vi "DefineScan.vi"() -> ()   [LabVIEW 2011]
doc: "Element for defineing the region to scan"
uses:
  <vilib>/vision/NI_Vision_Development_Module.lvlib
panel:
  out "Galvo pos i.image [m]":cluster{dbl, dbl}={0.005744, 0.00027999999999999987} {"?" format="%#_3p"; "?" format="%#_3p"}
  in  "Registerkarte":enum32{"scan", "view", "option"}(tab)
  in  "experiment":string="mysample_01"
  in  "pixels":cluster{"x-Pixel":i32, "y-Pixel":u16}={"x-Pixel"=400, "y-Pixel"=400} {"y-Pixel" min=2 max=4000 step=2; "x-Pixel" min=10 max=4000 step=1}
  in  "keep const.":u16(ring) items=["pix. size", "pixels"]
  in  "pixel size":cluster{dbl, dbl}={3e-07, 3e-07} {"?" min=0.0 max=0.01 step=5e-08 format="%#_4p"; "?" min=0.0 max=0.01 step=5e-08 format="%#_4p"}
  out "Turn loss %":dbl=0.5000000000000115 format="%#_4f"
  out "total time [s]":dbl=1.6 min=0.0005 step=0.001 format="%#_3f"
  in  "image size [m]":cluster{"x":dbl, "y":dbl}={"x"=0.00012, "y"=0.00012} {"y" min=0.0 max=0.01 step=1e-06 format="%#_4p"; "x" min=0.0 max=0.01 step=1e-06 format="%#_4p"}
  in  "Bidirektional":bool=TRUE
  in  "time [s]/point":dbl=1e-05 min=2.5e-07 step=1e-06 format="%#_3p"
  in  "ChangeScan":bool
  in  "Maximum":i32=97
  in  "Minimum":i32=3
  in  "Image loading method":bool=TRUE caption="Scan          calibration(new)"
  in  "Image to load":enum16{"marked", "last", "penultimate", "clear"}(ring)
  in  "scan to load":enum16{"marked", "last", "active"}(ring)=enum."last"
  in  "Galvo center [m] ii":cluster{dbl, dbl}={0.0002, -0.0008} {"?" min=-0.1 max=0.1 step=0.0001; "?" min=-0.1 max=0.1 step=0.0001}
  in  "LoadNewScan":bool
  in  "radius of view-x (6m)":dbl=0.006 min=0.0005 max=0.1 step=0.001
  in  "LoadNewImage":bool
  in  "Display Mapping Method":u32(ring)=16 items=["Default"=10, "Most Significant Bits"=11, "Full Dynamic"=12, "Downshift"=13, "Given Range"=14, "90% Dynamic"=15, "Given Percent Range"=16]
  in  "Image Oversampling":sgl=1.0 min=0.5 max=10 step=1
  in  "parabolic turn":bool=TRUE
  in  "times higher accelaration":dbl=1.0 min=1e-06 max=1000000.0 step=0.05
  in  "Transform":T1={"00 Pixel [m]"={-0.0058000000000000005, 0.0052}, "Rotate (rad)"=-0.0, "MirrorY"=TRUE, "pix/m"=41666.666666666664} caption="Pixel>Scan-i.image[m]" {"00 Pixel [m]"."?" format="%#_3p"; "00 Pixel [m]"."?" format="%#_3p"}
  in  "galvorotation (grad)":dbl=-0.0
  out "galvocycle":dbl=1e-05
  out "adclock":dbl=4000000.0
  in  "Objektive":dbl=60.0 format="%.1f"
  in  "SMdelay [Cycles]":i16=119
  in  "do not close at end":bool
  out "Image":T2(plugin-control)
  in  "Exit":bool
  # "m for 1E-3\nu for 1E-6\nn for 1E-9"
  # "all referenced to\nintermediate image\n!! so far no update: load new!"
  # "real position is \ni.image*Maginfication"
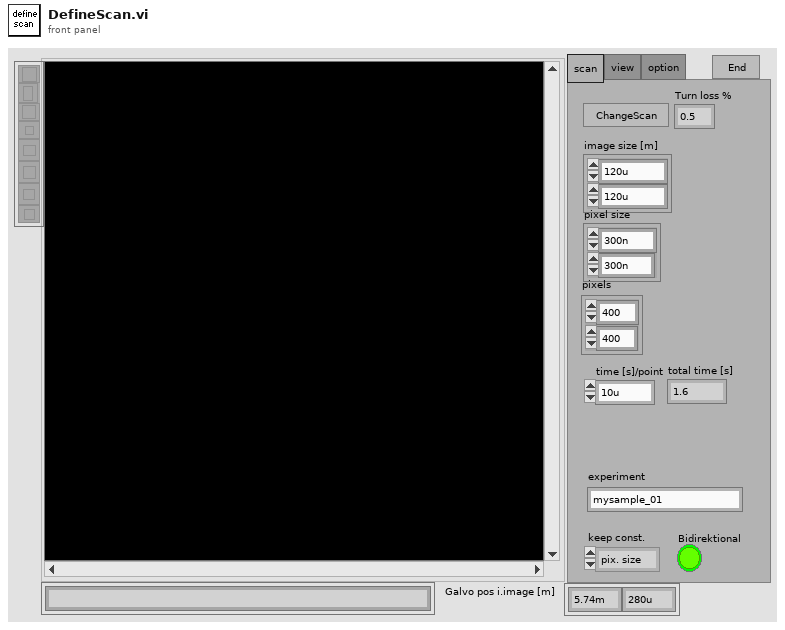
[diagram p1: front panel]
types:
  T1 = cluster{"00 Pixel [m]":cluster{dbl, dbl}, "Rotate (rad)":dbl, "MirrorY":bool, "pix/m":dbl}
  T2 = typedef "IMAQ Image.ctl" = refnum<image>
  T3 = cluster{"Pixel":i32, "Smartmovedelay [s]":dbl, "Loops":i32, "Bidirektional":bool, "SMCycle [s]":dbl, "AD-Frequency [Hz]":dbl, "Grad/m":dbl}
  T4 = typedef "Image Type" = u32
  T5 = enum16{"None/#Datasets", "Clear", "TagValueOf#", "AddValues", "ReadValue", "ChangeValue", "Get all"}
  T6 = cluster{"x Pixel":i32, "Lines":i32, "Bidirektional":bool, "AD-Frequency [Hz]":dbl, "Galvo Cycle [s]":dbl, "Galvodelay [s]":dbl, "max.accel. [m/s^2]":dbl}
  T7 = cluster{"Pixel":i32, "Smartmovedelay [s]":dbl, "lines":i32, "Bidirektional":bool, "SMCycle [s]":dbl, "AD-Frequency [Hz]":dbl, "Grad/m":dbl}
  T8 = cluster{"Zeit/Spirale (sync Pixel)":dbl, "Center":cluster{"x":dbl, "y":dbl}, "Radius":dbl}
  T9 = cluster{"Pixel on spiral":i32, "Smartmovedelay [s]":dbl, "lines":i32, "Bidirektional":bool, "SMCycle [s]":dbl, "AD-Frequency [Hz]":dbl, "Grad/m":dbl}
  T10 = typedef "Image Unit" = enum32{"Undefined", "Angström", "Micrometer", "Millimeter", "Centimeter", "Meter", "Kilometer", "Microinch", "Inch", "Feet", "Nautical miles", "Standard miles", "Steps"}
  T11 = enum16{"status", "createIMAQ", "getIMAQ", "getNumber", "deleteIMAQ", "deleteAll", "MemoryUsage", "GetAccess", "DecreaseAccess", "ActualIndex", "ElementToNumber"}
  T12 = enum16{"status", "saveMeta", "getMeta", "deleteMeta", "deleteAll", "MemoryUsage"}
  T13 = cluster{"Global Rectangle":i32[], "Contours":cluster{"Contour Type":u32, "ROI Type":u32, "Points":i32[]}[]}
  T14 = cluster{"Contour Type":u32, "ROI Type":u32, "Points":i32[]}[]
  T15 = cluster{"Contour Type":u32, "ROI Type":u32, "Points":i32[]}
  T16 = typedef "ScanControl.ctl" = cluster{"Time [s]":dbl, "action":T17, "channel":T18, "value (/s)":dbl}[]
  T17 = typedef "ScanControl_Action.ctl" = enum16{"Abs", "Rel", "Inc", "IncInc", "LoopStart", "LoopEnd", "WaitTriggerRising"}
  T18 = typedef "ScanControl_Channel.ctl" = enum16{"Com", "AnalogConfig", "AnalogValue", "GalvoX", "GalvoY", "Galvo3", "Galvo4", "Digital", "Free", "Loop", "SMoveTime", "Image1X", "Image1Y", "Image2X", "Image2Y"}
  T19 = cluster{"Global Rectangle[0]":i32, "Global Rectangle[1]":i32}
  T20 = cluster{"Point Out":cluster{dbl, dbl}, cluster{dbl, dbl}, cluster{dbl, dbl}, dbl}
  T21 = cluster{"Zeitpunkt [s]":dbl, "Wirkung":enum16{"Abs", "Rel", "Inc", "IncInc", "LoopStart", "LoopEnd"}, "Kanal":enum16{"Com", "AnalogConfig", "AnalogValue", "GalvoX", "GalvoY", "Galvo3", "Galvo4", "Digital", "Free", "Loop", "SMoveTime", "Image1X", "Image1Y", "Image2X", "Image2Y"}, "Wert (/s)":dbl}[]
  T22 = cluster{"fast/slow [m(ii)][0]":cluster{"x":dbl, "y":dbl}, "fast/slow [m(ii)][1]":cluster{"x":dbl, "y":dbl}}
  T23 = cluster{"number: 0 to 1":dbl, "number: 0 to 1":dbl}[]
  T24 = cluster{i32[], cluster{"Contour Type":u32, "ROI Type":u32, i32[]}[]}
  T25 = cluster{"Contour Type":u32, "ROI Type":u32, i32[]}[]
  T26 = cluster{"Contour Type":u32, "ROI Type":u32, i32[]}
  T27 = cluster{"Global Rectangle[0]":i32, "Global Rectangle[1]":i32, "Global Rectangle[2]":i32, "Global Rectangle[3]":i32}
  T28 = cluster{"Global Rectangle[2]":i32, "Global Rectangle[3]":i32}
  T29 = cluster{"Points[0]":i32, "Points[1]":i32, "Points[2]":i32, "Points[3]":i32, "Points[4]":i32}
  T30 = cluster{"Points[0]":i32, "Points[1]":i32, "Points[2]":i32, "Points[3]":i32}
  T31 = cluster{i32[], cluster{"Contour Type":u32, "ROI Type":u32, "Points":i32[]}[]}
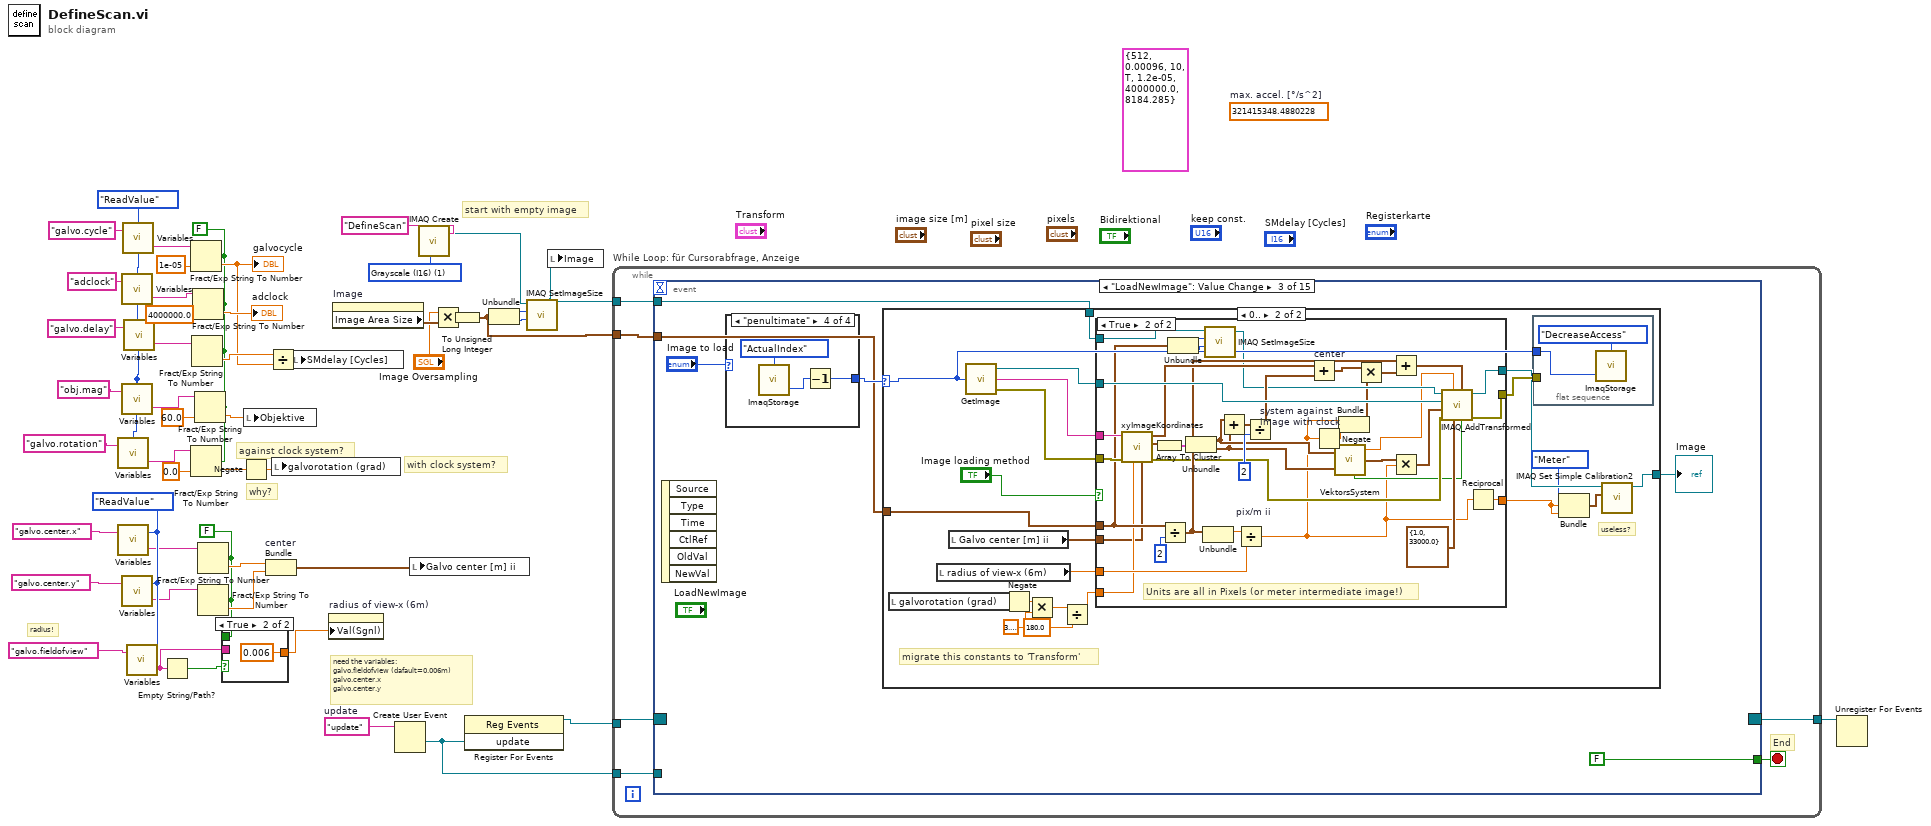
[diagram p0: block diagram]
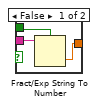
[diagram p2: hidden frame]
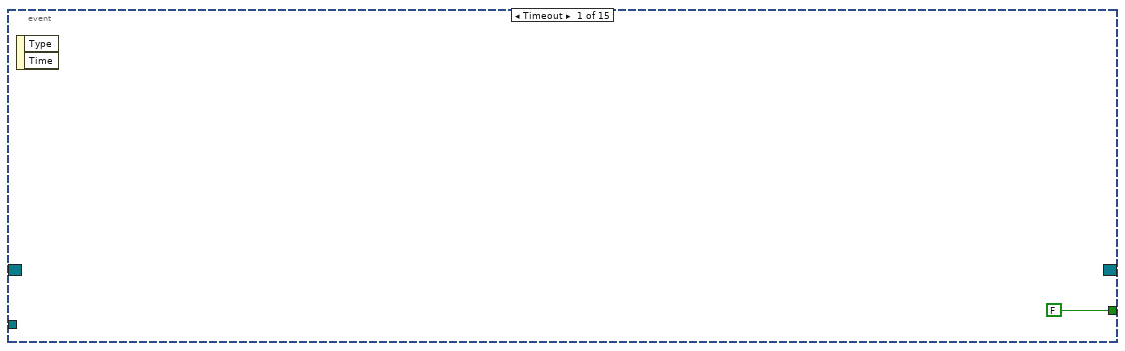
[diagram p3: hidden frame]
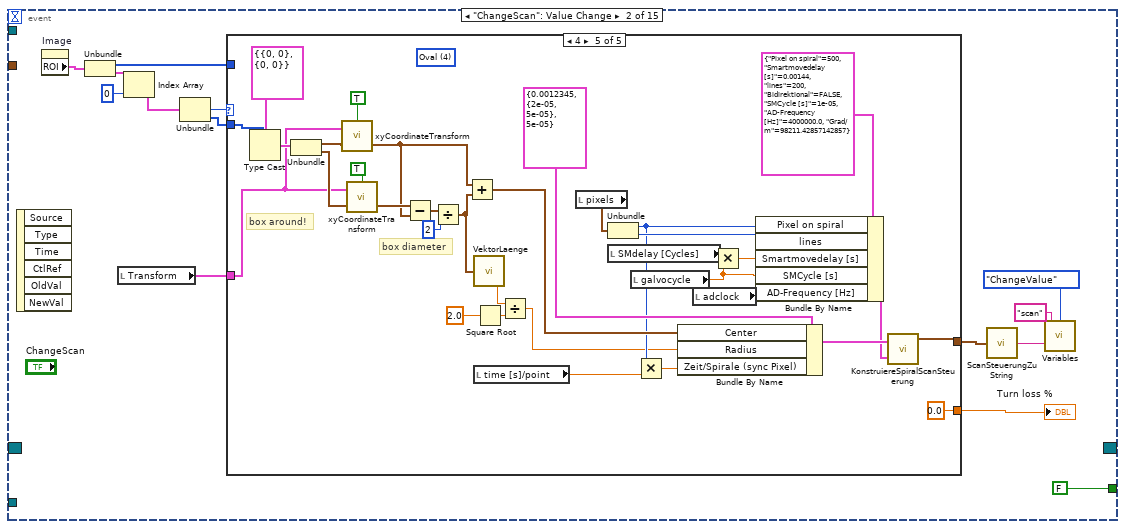
[diagram p4: hidden frame]
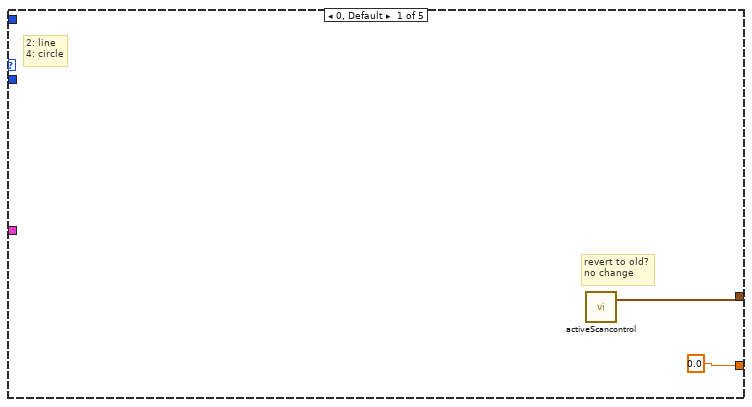
[diagram p5: hidden frame]
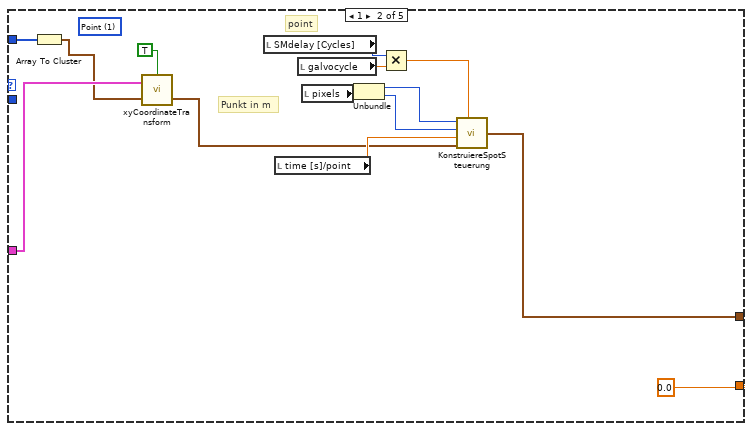
[diagram p6: hidden frame]
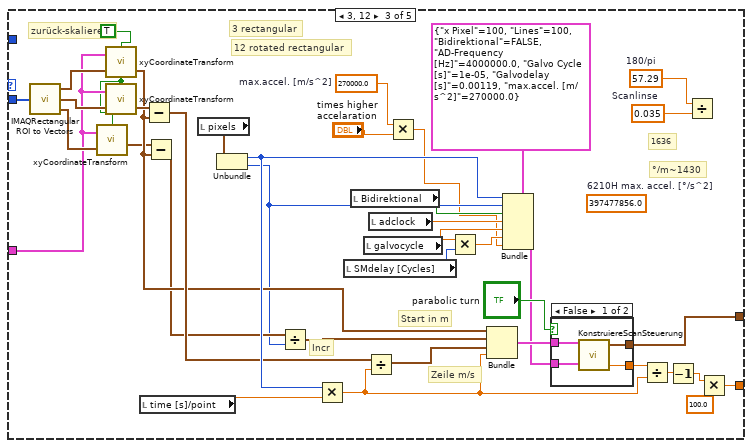
[diagram p7: hidden frame]
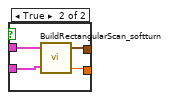
[diagram p8: hidden frame]
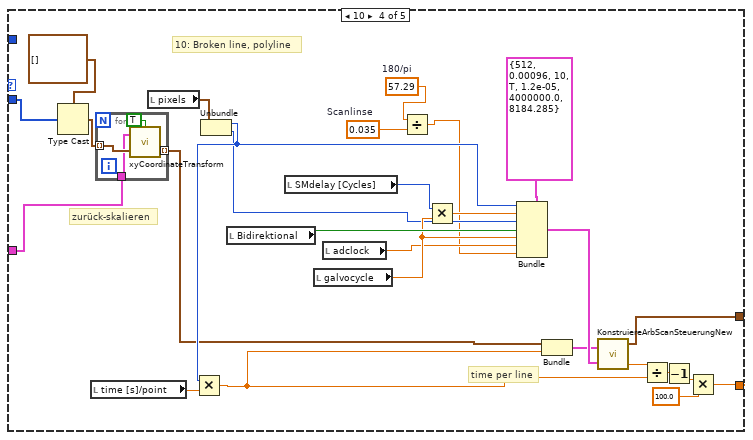
[diagram p9: hidden frame]
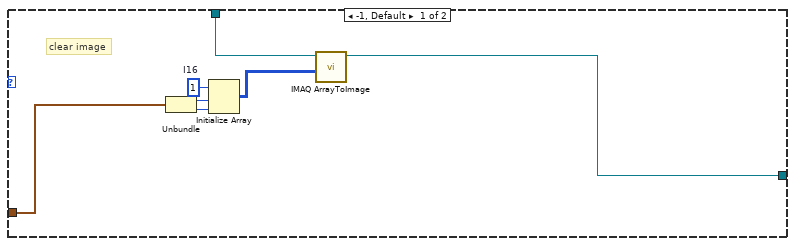
[diagram p10: hidden frame]
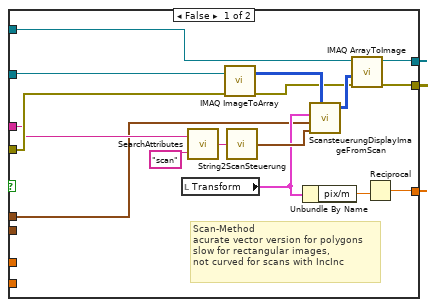
[diagram p11: hidden frame]
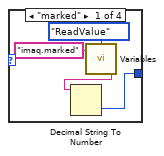
[diagram p12: hidden frame]
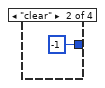
[diagram p13: hidden frame]
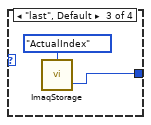
[diagram p14: hidden frame]
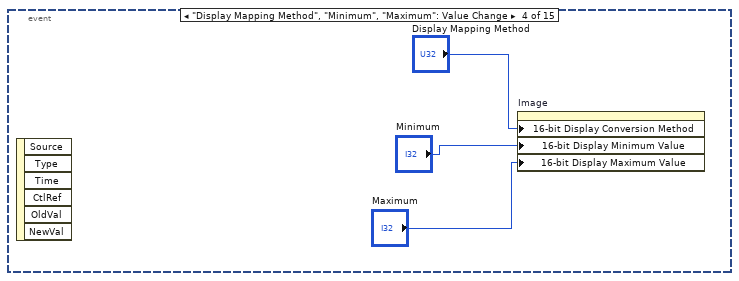
[diagram p15: hidden frame]
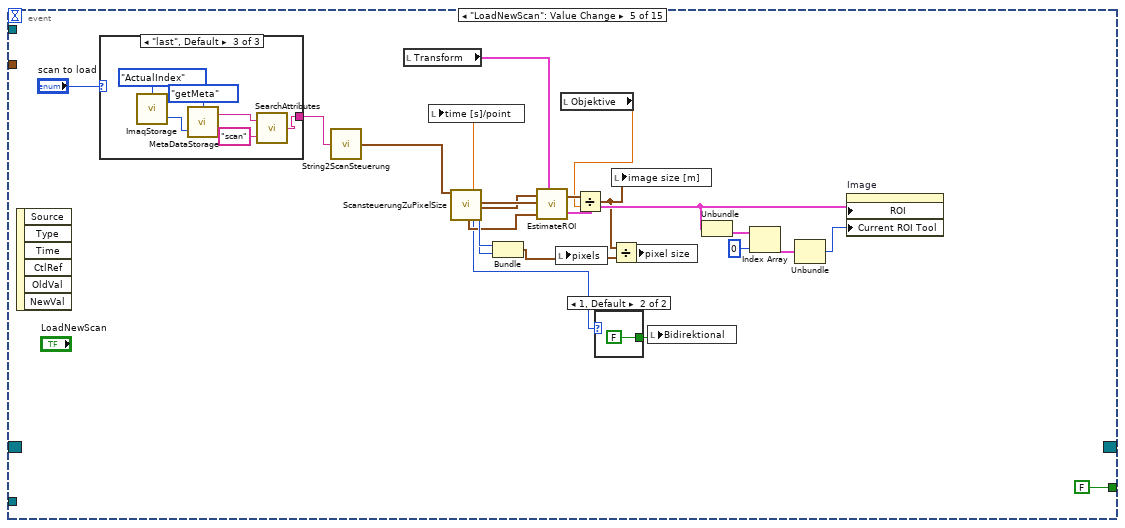
[diagram p16: hidden frame]
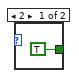
[diagram p17: hidden frame]
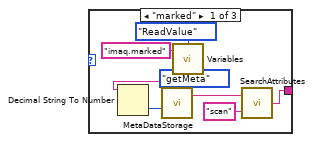
[diagram p18: hidden frame]
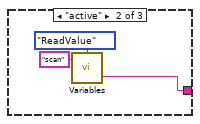
[diagram p19: hidden frame]
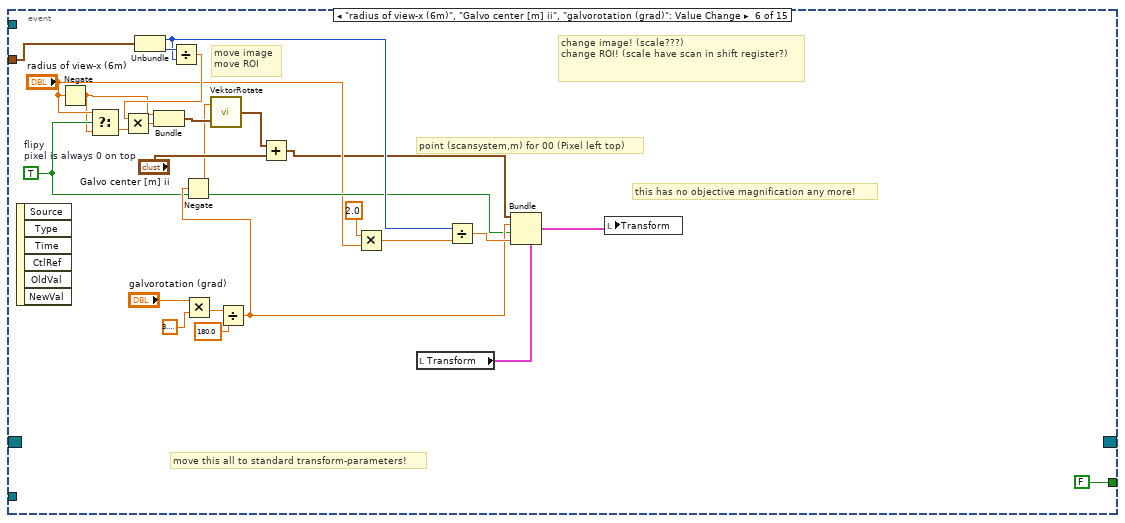
[diagram p20: hidden frame]
diagram:
  (unwired) 321415348.4880228  # max. accel. [°/s^2]
  (unwired) T3 {"Pixel"=512, "Smartmovedelay [s]"=0.00096, "Loops"=10, "Bidirektional"=TRUE, "SMCycle [s]"=1.2e-05, "AD-Frequency [Hz]"=4000000.0, "Grad/m"=8184.285} ("ParameterCluster")
  w10 = T4 1 items=["Grayscale (U8)", "Grayscale (I16)", "Grayscale (SGL)", "Complex (CSG)", "RGB (U32)", "HSL (U32)", "RGB (U64)", "Grayscale (U16)"] ("Image Type")
  w27 = FALSE ("use system decimal point (T)")
  w26 = T5."ReadValue" ("Command")
  w39 = "update"  # update
  w15 = FALSE ("use system decimal point (T)")
  w14 = T5."ReadValue" ("Command")
  # "against clock system?"
  # "with clock system?"
  # "why?"
  # "start with empty image"
  # "radius!"
  # "need the variables:\ngalvo.fieldofview (dafault=0.006m)\ngalvo.center.x\ngalvo.center.y"
  n1 = call "Variables.vi"("Tag in"="galvo.rotation", "Command"=w14) -> ("value out"=w17:string)  [unwired: 1 in, 2 out]
  n2 = call "Variables.vi"("Tag in"="galvo.center.x", "Command"=w26) -> ("value out"=w24:string)  [unwired: 1 in, 2 out]
  n3 = call "Variables.vi"("Tag in"="adclock", "Command"=w14) -> ("value out"=w47:string)  [unwired: 1 in, 2 out]
  n4 = call "Variables.vi"("Tag in"="obj.mag", "Command"=w14) -> ("value out"=w43:string)  [unwired: 1 in, 2 out]
  n5 = call "Variables.vi"("Tag in"="galvo.center.y", "Command"=w26) -> ("value out"=w23:string)  [unwired: 1 in, 2 out]
  n6 = call "Variables.vi"("Tag in"="galvo.cycle", "Command"=w14) -> ("value out"=w46:string)  [unwired: 1 in, 2 out]
  n7 = call "Variables.vi"("Tag in"="galvo.delay", "Command"=w14) -> ("value out"=w35:string)  [unwired: 1 in, 2 out]
  n8 = call "Variables.vi"("Tag in"="galvo.fieldofview", "Command"=w26) -> ("value out"=w30:string)  [unwired: 1 in, 2 out]
  n9 = Empty String/Path?(string/path=w30) -> (empty?=w31:bool)
  n10 = Fract/Exp String To Number(use system decimal point (T)=w15, string=w46, default (0 dbl)=1e-05 ("default (0 DBL)")) -> (number=w33:dbl)  [unwired: 2 out]
  "galvocycle" <- w33
  n11 = Fract/Exp String To Number(use system decimal point (T)=w15, string=w17, default (0 dbl)=0.0 ("default (0 DBL)")) -> (number=w13:dbl)  [unwired: 2 out]
  n12 = Fract/Exp String To Number(use system decimal point (T)=w15, string=w35) -> (number=w34:dbl)  [unwired: 3 out]
  n13 = Fract/Exp String To Number(use system decimal point (T)=w15, string=w47, default (0 dbl)=4000000.0 ("default (0 DBL)")) -> (number=→"adclock":dbl)  [unwired: 2 out]
  n14 = Fract/Exp String To Number(use system decimal point (T)=w15, string=w43, default (0 dbl)=60.0 ("default (0 DBL)")) -> (number=w20:dbl)  [unwired: 2 out]
  n15 = Fract/Exp String To Number(use system decimal point (T)=w27, string=w24) -> (number=w28:dbl)  [unwired: 3 out]
  n16 = Fract/Exp String To Number(use system decimal point (T)=w27, string=w23) -> (number=w29:dbl)  [unwired: 3 out]
  n17 = case shown="True" w31 {
    tunnel: w30 -> [w53 _]
    tunnel: w27 -> [w52 _]
    tunnel: [w51 0.006] -> w11
    frame False {
      n18 = Fract/Exp String To Number(use system decimal point (T)=w52, string=w53) -> (number=w51:dbl)  [unwired: 3 out]
    }
    frame True {
    }
  }
  n19 = Negate(x=w13) -> (-x=w12:dbl)
  n20 = local write "Objektive"(w20) -> ()
  n21 = Bundle "center"(w28, w29) -> (w19:cluster{dbl, dbl})  [unwired: 1 out]
  n22 = Divide(x=w34, y=w33) -> (x/y=w32:dbl)
  n23 = local write "galvorotation (grad)"(w12) -> ()
  n24 = local write "SMdelay [Cycles]"(w32) -> ()
  n25 = property on="radius of view-x (6m)" class="DigNum (strict)"("Val(Sgnl)"=w11) -> ()  [unwired: 2 in, 2 out]
  n26 = property on="Image" class="ImageControl"() -> ("Image Area Size"=w6:cluster{"Width":u32, "Height":u32})  [unwired: 2 in, 2 out]
  n27 = Create User Event(user event datatype=w39) -> (user event=w36:refnum<user-event>)  [unwired: 1 in, 1 out]
  n28 = local write "Galvo center [m] ii"(w19) -> ()
  n29 = call "IMAQ Create"("Image Name"="DefineScan", "Image Type"=w10) -> ("New Image"=w5:T2)  [unwired: 2 in, 2 out]
  n30 = Multiply(x="Image Oversampling", y=w6) -> (x*y=w3:cluster{"Width":sgl, "Height":sgl})
  n31 = To Unsigned Long Integer(number=w3) -> (unsigned 32bit integer=w1:cluster{"Width":u32, "Height":u32})
  n32 = register-events(w36) -> (reference out=w38:refnum<event-registration>)  [unwired: 2 in, 1 out]
  n33 = Unbundle(w1) -> ("Width"=w8:u32, "Height"=w7:u32)
  n34 = call "IMAQ SetImageSize"("Y Resolution"=w7, "X Resolution"=w8, "Image"=w5) -> ("Image Out"=w4:T2)  [unwired: 1 in, 2 out]
  n35 = local write "Image"(w4) -> ()
  n36 = while "While Loop: für Cursorabfrage, Anzeige" {
    tunnel: w38 -> [w59]
    tunnel: [w58] -> w37
    tunnel: w36 -> [w57]
    tunnel: w4 -> [w56]
    tunnel: w1 -> [w55]
    stop <- w60 stop-if-true
    # "End"
    n37 = event shown="[2] \"LoadNewImage\": Value Change" {
      selector: w59 -> [_ _ _ _ _ _ _ _ _ _ _ _ _ _ _]
      dyn-events: [_ _ _ _ _ _ _ _ _ _ _ _ _ _ _] -> w58
      timeout: _ -> [_ _ _ _ _ _ _ _ _ _ _ _ _ _ _]
      tunnel: [FALSE FALSE FALSE _ FALSE ("Exit") FALSE ("Exit") FALSE ("Exit") FALSE ("Exit") _ FALSE ("Exit") FALSE ("Exit") FALSE ("Exit") _ "Exit" FALSE] -> w60
      tunnel: w57 -> [_ _ _ _ _ _ _ w385 _ w403 w501 w521 _ _ _]
      tunnel: w56 -> [_ _ w205 _ _ _ _ _ _ _ _ _ _ _ _]
      tunnel: w55 -> [_ _ w202 _ _ w346 _ _ _ _ _ _ _ _ _]
      event Timeout {
        n38 = event-data() -> ()  [unwired: 3 out]
      }
      event "ChangeScan": Value Change {
        n39 = event-data() -> ()  [unwired: 7 out]
        n40 = property on="Image" class="ImageControl"() -> ("ROI"=w74:T13)  [unwired: 2 in, 2 out]
        n41 = Unbundle(w74) -> ("Global Rectangle"=w73:i32[], "Contours"=w72:T14)
        n42 = local read "Transform"() -> (w62:T1)
        n43 = Index Array(array=w72, index=0) -> (element=w70:T15)
        n44 = Unbundle(w70) -> ("ROI Type"=w69:u32, "Points"=w68:i32[])  [unwired: 1 out]
        n45 = case shown="4" w69 {
          tunnel: w73 -> [_ w90 _ _ _]
          tunnel: w68 -> [_ _ w126 w147 w197]
          tunnel: [w77 w87 w118 w151 w201] -> w67
          tunnel: [0.0 0.0 w117 w146 0.0] -> w63
          tunnel: w62 -> [_ w80 w106 w141 w179]
          frame 0, Default {
            # "2: line\n4: circle"
            # "revert to old?\nno change"
            n46 = call "activeScancontrol.vi"() -> ("ScanSteuerung"=w77:T16)  [unwired: 2 in, 1 out]
          }
          frame 1 {
            (unwired) u32 1 items=["No Selection", "Point", "Line", "Rectangle", "Oval", "Polygon", "Free", "Annulus", "Unused2", "Unused3", "Broken Line", "Free Hand Line", "Rotated Rectangle"] ("Type")
            # "Punkt in m"
            # "point"
            n47 = Array To Cluster(array=w90) -> (cluster=w79:T19)
            n48 = call "xyCoordinateTransform.vi"("Point in"=w79, "Transform (Center first)"=w80, "Back"=TRUE) -> ("Point Out"=w78:cluster{dbl, dbl})  [unwired: 2 out]
            n49 = local read "SMdelay [Cycles]"() -> (w91:i16)
            n50 = local read "time [s]/point"() -> (w88:dbl)
            n51 = local read "galvocycle"() -> (w86:dbl)
            n52 = local read "pixels"() -> (w84:cluster{"x-Pixel":i32, "y-Pixel":u16})
            n53 = Unbundle(w84) -> ("x-Pixel"=w83:i32, "y-Pixel"=w82:u16)
            n54 = Multiply(x=w91, y=w86) -> (x*y=w89:dbl)
            n55 = call "KonstruiereSpotSteuerung.vi"("SMtime"=w89, "Punkt [m]"=w78, "Time [s]/Point"=w88, "y-Pixel"=w82, "x-Pixel"=w83) -> ("ScanSteuerung"=w87:T16)  [unwired: 1 out]
          }
          frame 3, 12 {
            w94 = 270000.0  # max.accel. [m/s^2]
            (unwired) 397477856.0  # 6210H max. accel. [°/s^2]
            w105 = TRUE ("Back")
            w104 = 57.29  # 180/pi
            w129 = 0.035  # Scanlinse
            # "°/m~1430"
            # "1636"
            # "3 rectangular"
            # "12 rotated rectangular"
            # "Start in m"
            # "zurück-skalieren"
            # "Zeile m/s"
            # "Incr"
            n56 = call "IMAQRectangularROI to Vectors.vi"("Array"=w126) -> ("Start"=w114:cluster{"x":dbl, "y":dbl}, "fast end"=w113:cluster{"x":dbl, "y":dbl}, "slow end"=w111:cluster{"x":dbl, "y":dbl})
            n57 = call "xyCoordinateTransform.vi"("Point in"=w111, "Transform (Center first)"=w106, "Back"=w105) -> ("Point Out"=w108:cluster{dbl, dbl})  [unwired: 2 out]
            n58 = call "xyCoordinateTransform.vi"("Point in"=w114, "Transform (Center first)"=w106, "Back"=w105) -> ("Point Out"=w109:cluster{dbl, dbl})  [unwired: 2 out]
            n59 = call "xyCoordinateTransform.vi"("Point in"=w113, "Transform (Center first)"=w106, "Back"=w105) -> ("Point Out"=w110:cluster{dbl, dbl})  [unwired: 2 out]
            n60 = local read "time [s]/point"() -> (w127:dbl)
            n61 = Subtract(x=w110, y=w109) -> (x-y=w112:cluster{dbl, dbl})
            n62 = Subtract(x=w108, y=w109) -> (x-y=w107:cluster{dbl, dbl})
            n63 = local read "pixels"() -> (w116:cluster{"x-Pixel":i32, "y-Pixel":u16})
            n64 = Unbundle(w116) -> ("x-Pixel"=w115:i32, "y-Pixel"=w100:u16)
            n65 = Divide(x=w107, y=w100) -> (x/y=w125:cluster{dbl, dbl})
            n66 = Multiply(x=w115, y=w127) -> (x*y=w122:dbl)
            n67 = local read "SMdelay [Cycles]"() -> (w95:i16)
            n68 = local read "Bidirektional"() -> (w99:bool)
            n69 = local read "galvocycle"() -> (w96:dbl)
            n70 = Divide(x=w112, y=w122) -> (x/y=w124:cluster{dbl, dbl})
            n71 = local read "adclock"() -> (w98:dbl)
            n72 = Multiply(x=w94, y="times higher accelaration") -> (x*y=w92:dbl)
            n73 = Multiply(x=w96, y=w95) -> (x*y=w97:dbl)
            n74 = Bundle("Point Out"=w109, w125, w124, w122) -> (w128:T20)  [unwired: 1 out]
            n75 = Bundle(cluster=T6 {"x Pixel"=100, "Lines"=100, "Bidirektional"=FALSE, "AD-Frequency [Hz]"=4000000.0, "Galvo Cycle [s]"=1e-05, "Galvodelay [s]"=0.00119, "max.accel. [m/s^2]"=270000.0} ("ParameterCluster"), "x Pixel"=w115, "Lines"=w100, "Bidirektional"=w99, "AD-Frequency [Hz]"=w98, "Galvo Cycle [s]"=w96, "Galvodelay [s]"=w97, "max.accel. [m/s^2]"=w92) -> (w101:T6)
            n76 = case shown="False" "parabolic turn" {
              tunnel: w128 -> [w133 w137]
              tunnel: [w132 w135] -> w123
              tunnel: [w131 w136] -> w118
              tunnel: w101 -> [w130 w134]
              frame False {
                n77 = call "KonstruiereScanSteuerung.vi"("VektorCluster"=w133, "ParameterCluster"=w130) -> ("ScanSteuerung"=w131:T21, "Line+Turn [s]"=w132:dbl)  [unwired: 1 out]
              }
              frame True {
                n78 = call "BuildRectangularScan_softturn.vi"("VektorCluster"=w137, "ParameterCluster"=w134) -> ("ScanSteuerung"=w136:T21, "Line+Turn [s]"=w135:dbl)  [unwired: 1 out]
              }
            }
            n79 = Divide(x=w123, y=w122) -> (x/y=w121:dbl)
            n80 = Decrement(x=w121) -> (x-1=w120:dbl)
            n81 = Divide(x=w104, y=w129) -> ()  [unwired: 1 out]
            n82 = Multiply(x=w120, y=100.0) -> (x*y=w117:dbl)
          }
          frame 10 {
            w139 = 57.29  # 180/pi
            w162 = 0.035  # Scanlinse
            # "10: Broken line, polyline"
            # "zurück-skalieren"
            # "time per line"
            n83 = Type Cast(type=cluster{i32, i32}[] [], x=w147) -> (*(type *) &x=w142:cluster{i32, i32}[])
            n84 = local read "time [s]/point"() -> (w157:dbl)
            n85 = for {
              tunnel: w142 -> [w168] mode=indexing
              tunnel: w141 -> [w167]
              tunnel: [w166] -> w140 mode=indexing
              n86 = call "xyCoordinateTransform.vi"("Point in"=w168, "Transform (Center first)"=w167, "Back"=TRUE) -> ("Point Out"=w166:cluster{dbl, dbl})  [unwired: 2 out]
            }
            n87 = local read "pixels"() -> (w145:cluster{"x-Pixel":i32, "y-Pixel":u16})
            n88 = Unbundle(w145) -> ("x-Pixel"=w144:i32, "y-Pixel"=w143:u16)
            n89 = Multiply(x=w144, y=w157) -> (x*y=w155:dbl)
            n90 = local read "Bidirektional"() -> (w158:bool)
            n91 = local read "SMdelay [Cycles]"() -> (w159:i16)
            n92 = local read "galvocycle"() -> (w150:dbl)
            n93 = local read "adclock"() -> (w149:dbl)
            n94 = Divide(x=w139, y=w162) -> (x/y=w138:dbl)
            n95 = Multiply(x=w159, y=w150) -> (x*y=w164:dbl)
            n96 = Bundle(cluster=T7 {"Pixel"=512, "Smartmovedelay [s]"=0.00096, "lines"=10, "Bidirektional"=TRUE, "SMCycle [s]"=1.2e-05, "AD-Frequency [Hz]"=4000000.0, "Grad/m"=8184.285} ("ParameterCluster"), "Pixel"=w144, "Smartmovedelay [s]"=w164, "lines"=w143, "Bidirektional"=w158, "SMCycle [s]"=w150, "AD-Frequency [Hz]"=w149, "Grad/m"=w138) -> (w161:T7)
            n97 = Bundle(w140, w155) -> (w160:cluster{cluster{dbl, dbl}[], dbl})  [unwired: 1 out]
            n98 = call "KonstruiereArbScanSteuerungNew.vi"("VektorCluster"=w160, "ParameterCluster"=w161) -> ("ScanSteuerung"=w151:T21, "Line+Turn [s]"=w156:dbl)  [unwired: 1 out]
            n99 = Divide(x=w156, y=w155) -> (x/y=w154:dbl)
            n100 = Decrement(x=w154) -> (x-1=w153:dbl)
            n101 = Multiply(x=w153, y=100.0) -> (x*y=w146:dbl)
          }
          frame 4 {
            (unwired) u32 4 items=["No Selection", "Point", "Line", "Rectangle", "Oval", "Polygon", "Free", "Annulus", "Unused2", "Unused3", "Broken Line", "Free Hand Line", "Rotated Rectangle"] ("Type")
            # "box diameter"
            # "box around!"
            n102 = Type Cast(type=cluster{cluster{i32, i32}, cluster{i32, i32}} {{0, 0}, {0, 0}}, x=w197) -> (*(type *) &x=w195:cluster{cluster{i32, i32}, cluster{i32, i32}})
            n103 = Unbundle(w195) -> (w182:cluster{i32, i32}, w184:cluster{i32, i32})
            n104 = call "xyCoordinateTransform.vi"("Point in"=w182, "Transform (Center first)"=w179, "Back"=TRUE) -> ("Point Out"=w181:cluster{dbl, dbl})  [unwired: 2 out]
            n105 = call "xyCoordinateTransform.vi"("Point in"=w184, "Transform (Center first)"=w179, "Back"=TRUE) -> ("Point Out"=w183:cluster{dbl, dbl})  [unwired: 2 out]
            n106 = Subtract(x=w183, y=w181) -> (x-y=w194:cluster{dbl, dbl})
            n107 = Divide(x=w194, y=2) -> (x/y=w173:cluster{dbl, dbl})
            n108 = Add(x=w181, y=w173) -> (x+y=w180:cluster{dbl, dbl})
            n109 = call "VektorLaenge.vi"("Vektor"=w173) -> ("Vektorlänge"=w172:dbl)
            n110 = local read "time [s]/point"() -> (w177:dbl)
            n111 = Square Root(x=2.0) -> (sqrt(x)=w170:dbl)
            n112 = Divide(x=w172, y=w170) -> (x/y=w169:dbl)
            n113 = local read "pixels"() -> (w191:cluster{"x-Pixel":i32, "y-Pixel":u16})
            n114 = Unbundle(w191) -> ("x-Pixel"=w176:i32, "y-Pixel"=w189:u16)
            n115 = local read "SMdelay [Cycles]"() -> (w188:i16)
            n116 = local read "galvocycle"() -> (w175:dbl)
            n117 = Multiply(x=w176, y=w177) -> (x*y=w178:dbl)
            n118 = Bundle By Name(cluster=T8 {"Zeit/Spirale (sync Pixel)"=0.0012345, "Center"={"x"=2e-05, "y"=5e-05}, "Radius"=5e-05} ("VektorCluster"), "Center"=w180, "Radius"=w169, "Zeit/Spirale (sync Pixel)"=w178) -> (w192:T8)
            n119 = local read "adclock"() -> (w174:dbl)
            n120 = Multiply(x=w188, y=w175) -> (x*y=w187:dbl)
            n121 = Bundle By Name(cluster=T9 {"Pixel on spiral"=500, "Smartmovedelay [s]"=0.00144, "lines"=200, "Bidirektional"=FALSE, "SMCycle [s]"=1e-05, "AD-Frequency [Hz]"=4000000.0, "Grad/m"=98211.42857142857} ("ParameterCluster"), "Pixel on spiral"=w176, "lines"=w189, "Smartmovedelay [s]"=w187, "SMCycle [s]"=w175, "AD-Frequency [Hz]"=w174) -> (w190:T9)
            n122 = call "KonstruiereSpiralScanSteuerung.vi"("VektorCluster"=w192, "ParameterCluster"=w190) -> ("ScanSteuerung"=w201:T21)  [unwired: 2 out]
          }
        }
        "Turn loss %" <- w63
        n123 = call "ScanSteuerungZuString.vi"("ScanSteuerung neu"=w67) -> ("String"=w64:string)
        n124 = call "Variables.vi"("value"=w64, "Tag in"="scan" ("Name"), "Command"=T5."ChangeValue") -> ()  [unwired: 3 out]
      }
      event "LoadNewImage": Value Change {
        n125 = event-data() -> ()  [unwired: 7 out]
        n126 = case shown="\"penultimate\"" "Image to load" {
          tunnel: [w291 -1 ("Number out") w297 w298] -> w203
          frame "marked" {
            n127 = call "Variables.vi"("Tag in"="imaq.marked", "Command"=T5."ReadValue") -> ("value out"=w292:string)  [unwired: 1 in, 2 out]
            n128 = Decimal String To Number(string=w292) -> (number=w291:i32)  [unwired: 3 out]
          }
          frame "clear" {
          }
          frame "last", Default {
            n129 = call "ImaqStorage.vi"("Command"=T11."ActualIndex") -> ("Number out"=w297:i32)  [unwired: 2 in, 1 out]
          }
          frame "penultimate" {
            n130 = call "ImaqStorage.vi"("Command"=T11."ActualIndex") -> ("Number out"=w300:i32)  [unwired: 2 in, 1 out]
            n131 = Decrement(x=w300) -> (x-1=w298:i32)
          }
        }
        n132 = case shown="0.." w203 {
          selector: w203 -> [_ w221]
          tunnel: [w213 w218] -> w206
          tunnel: w205 -> [w214 w230]
          tunnel: w202 -> [w212 w220]
          frame -1, Default {
            w209 = i16 1  # I16
            # "clear image"
            n133 = Unbundle(w212) -> ("Width"=w211:u32, "Height"=w210:u32)
            n134 = Initialize Array(w209, w211, w210) -> (w208:i16[][])
            n135 = call "IMAQ ArrayToImage"("Image Pixels (I16)"=w208, "Image"=w214) -> ("Image Out"=w213:T2)  [unwired: 4 in, 5 out]
          }
          frame 0.. {
            # "migrate this constants to 'Transform'"
            # "useless?"
            n136 = local read "galvorotation (grad)"() -> (w227:dbl)
            n137 = local read "radius of view-x (6m)"() -> (w231:dbl)
            n138 = local read "Galvo center [m] ii"() -> (w223:cluster{dbl, dbl})
            n139 = call "GetImage.vi"("Image Number"=w221) -> ("Image"=w235:T2, "string"=w233:string, "error out"=w234:errorcluster)  [unwired: 1 out]
            n140 = Negate(x=w227) -> (-x=w222:dbl)
            n141 = Multiply(x=w222, y=3.141592653589793) -> (x*y=w228:dbl)
            n142 = Divide(x=w228, y=180.0) -> (x/y=w224:dbl)
            n143 = case shown="True" "Image loading method" {
              tunnel: w235 -> [w239 w288]
              tunnel: [w241 w287] -> w219
              tunnel: w234 -> [w238 w286]
              tunnel: [w243 w253] -> w215
              tunnel: w233 -> [w237 w285]
              tunnel: [w242 w284] -> w232
              tunnel: w231 -> [_ w283]
              tunnel: w220 -> [w236 w282]
              tunnel: w230 -> [w240 w281]
              tunnel: w224 -> [_ w260]
              tunnel: w223 -> [_ w259]
              frame False {
                # "Scan-Method\nacurate vector version for polygons\nslow for rectangular images,\nnot curved for scans with IncInc"
                n144 = local read "Transform"() -> (w246:T1)
                n145 = call "SearchAttributes.vi"("Search"="scan", "String"=w237) -> ("ValueText"=w251:string)
                n146 = call "IMAQ ImageToArray"("error in (no error)"=w238, "Image"=w239) -> ("error out"=w244:errorcluster, "Image Pixels (I16)"=w249:i16[][])  [unwired: 1 in, 4 out]
                n147 = call "String2ScanSteuerung.vi"("String"=w251) -> ("ScanSteuerung"=w248:T16)
                n148 = Unbundle By Name(w246) -> ("pix/m"=w245:dbl)
                n149 = call "ScansteuerungDisplayImageFromScan.vi"("Transform (Center first)"=w246, "Imagesize [Pixel]"=w236, "ScanSteuerung"=w248, "Intensity Graph"=w249) -> ("PixmapBild"=w247:i16[][])  [unwired: 3 out]
                n150 = call "IMAQ ArrayToImage"("error in (no error)"=w244, "Image Pixels (I16)"=w247, "Image"=w240) -> ("error out"=w242:errorcluster, "Image Out"=w241:T2)  [unwired: 3 in, 4 out]
                n151 = Reciprocal(x=w245) -> (1/x=w243:dbl)
              }
              frame True {
                # "Units are all in Pixels (or meter intermediate image!)"
                n152 = call "xyImageKoordinates.vi"("Galvo.center ii"=w259, "GalvoScanRotation [rad]"=w260, "error in (no error)"=w286, "String"=w285) -> ("error out"=w266:errorcluster, "fast/slow [m(ii)]"=w277:cluster{"x":dbl, "y":dbl}[], "start [m(ii)] (without stage)"=w273:cluster{dbl, dbl})  [unwired: 5 out]
                n153 = Array To Cluster(array=w277) -> (cluster=w276:T22)
                n154 = Divide(x=w282, y=2) -> (x/y=w269:cluster{"Width":dbl, "Height":dbl})
                n155 = Unbundle(w282) -> ("Width"=w264:u32, "Height"=w263:u32)
                n156 = Unbundle(w276) -> ("fast/slow [m(ii)][0]"=w258:cluster{"x":dbl, "y":dbl}, "fast/slow [m(ii)][1]"=w257:cluster{"x":dbl, "y":dbl})
                n157 = Unbundle(w269) -> ("Width"=w278:dbl)  [unwired: 1 out]
                n158 = call "IMAQ SetImageSize"("Y Resolution"=w263, "X Resolution"=w264, "Image"=w281) -> ("Image Out"=w265:T2)  [unwired: 1 in, 2 out]
                n159 = Add(x=w258, y=w257) -> (x+y=w275:cluster{"x":dbl, "y":dbl})
                n160 = Divide "pix/m ii"(x=w278, y=w283) -> (x/y=w252:dbl)
                n161 = Divide(x=w275, y=2) -> (x/y=w272:cluster{"x":dbl, "y":dbl})
                n162 = Add "center"(x=w273, y=w272) -> (x+y=w271:cluster{dbl, dbl})
                n163 = Negate "system against\nimage with clock"(x=w252) -> (-x=w262:dbl)
                n164 = call "VektorsSystem.vi"("x-Vector"=w258, "y-Vector"=w257) -> ("x-Vector Angle [degrees]"=w255:dbl, "Vector length"=w256:cluster{"x":dbl, "y":dbl}, "against clock = true"=w254:bool)  [unwired: 1 out]
                n165 = Bundle(w252, w262) -> (w261:cluster{dbl, dbl})  [unwired: 1 out]
                n166 = Multiply(x=w271, y=w261) -> (x*y=w270:cluster{dbl, dbl})
                n167 = Add(x=w269, y=w270) -> (x+y=w268:cluster{dbl, dbl})
                n168 = Multiply(x=w256, y=w252) -> (x*y=w267:cluster{"x":dbl, "y":dbl})
                n169 = call "IMAQ_AddTransformed.vi"("flip y"=w254, "center(0,0 = left,top)"=w268, "Range to display"=cluster{"Lower value":sgl, "Upper value":sgl} {"Lower value"=1.0, "Upper value"=33000.0}, "Angle (degrees)"=w255, "error in (no error)"=w266, "New Pixel Size"=w267, "Image to place in"=w288, "Image Src (Large)"=w265) -> ("error out"=w284:errorcluster, "Image Dst Out"=w287:T2)  [unwired: 2 out]
                n170 = Reciprocal(x=w252) -> (1/x=w253:dbl)
              }
            }
            n171 = flat-sequence {
              tunnel: w221 -> [w289]
              tunnel: w232 -> [_]
              frame #0 {
                n172 = call "ImaqStorage.vi"("Number"=w289, "Command"=T11."DecreaseAccess") -> ()  [unwired: 1 in, 2 out]
              }
            }
            n173 = Bundle("Unit"=Image_Unit."Meter", w215, w215) -> (w217:cluster{"Unit":T10, dbl, dbl})  [unwired: 1 in]
            n174 = call "IMAQ Set Simple Calibration2"("Pixel Distances"=w217, "Image"=w219) -> ("Calibration Template Image"=w218:T2)  [unwired: 8 in, 1 out]
          }
        }
        "Image" <- w206
      }
      event "Display Mapping Method", "Minimum", "Maximum": Value Change {
        n175 = event-data() -> ()  [unwired: 7 out]
        n176 = property on="Image" class="ImageControl"("16-bit Display Conversion Method"="Display Mapping Method", "16-bit Display Minimum Value"="Minimum", "16-bit Display Maximum Value"="Maximum") -> ()  [unwired: 2 in, 2 out]
      }
      event "LoadNewScan": Value Change {
        n177 = event-data() -> ()  [unwired: 7 out]
        n178 = case shown="\"last\", Default" "scan to load" {
          tunnel: [w329 w337 w340] -> w306
          frame "marked" {
            n179 = call "Variables.vi"("Tag in"="imaq.marked", "Command"=T5."ReadValue") -> ("value out"=w334:string)  [unwired: 1 in, 2 out]
            n180 = Decimal String To Number(string=w334) -> (number=w332:i32)  [unwired: 3 out]
            n181 = call "MetaDataStorage.vi"("Number"=w332, "Command"=T12."getMeta") -> ("Mata out"=w331:string)  [unwired: 1 in, 1 out]
            n182 = call "SearchAttributes.vi"("Search"="scan", "String"=w331) -> ("ValueText"=w329:string)
          }
          frame "active" {
            n183 = call "Variables.vi"("Tag in"="scan", "Command"=T5."ReadValue") -> ("value out"=w337:string)  [unwired: 1 in, 2 out]
          }
          frame "last", Default {
            n184 = call "ImaqStorage.vi"("Command"=T11."ActualIndex") -> ("Number out"=w343:i32)  [unwired: 2 in, 1 out]
            n185 = call "MetaDataStorage.vi"("Number"=w343, "Command"=T12."getMeta") -> ("Mata out"=w341:string)  [unwired: 1 in, 1 out]
            n186 = call "SearchAttributes.vi"("Search"="scan", "String"=w341) -> ("ValueText"=w340:string)
          }
        }
        n187 = call "String2ScanSteuerung.vi"("String"=w306) -> ("ScanSteuerung"=w317:T16)
        n188 = local read "Transform"() -> (w308:T1)
        n189 = call "ScansteuerungZuPixelSize.vi"("ScanSteuerung"=w317) -> ("Galvo one path"=w320:T23, "Pixeltime in s"=w326:dbl, "Lines/loop"=w315:i16, "yPixel"=w324:i32, "xpixel"=w325:i32, "Slow-Vektors"=w321:cluster{"meter":dbl, "meter":dbl}, "last-fast-vektor (exact)"=w318:cluster{"meter":dbl, "meter":dbl})  [unwired: 1 in, 11 out]
        n190 = local write "time [s]/point"(w326) -> ()
        n191 = Bundle("xpixel"=w325, "yPixel"=w324) -> (w323:cluster{"xpixel":i32, "yPixel":i32})  [unwired: 1 out]
        n192 = call "EstimateROI.vi"("Fast-Vektor (exaxt)"=w318, "Transform m->Pix  (Center first)"=w308, "Slow-Vektors"=w321, "Galvo one path"=w320) -> ("image size"=w319:cluster{"x":dbl, "y":dbl}, "ROI"=w314:T24)  [unwired: 1 in]
        n193 = local write "pixels"(w323) -> ()
        n194 = local read "Objektive"() -> (w304:dbl)
        n195 = Divide(x=w319, y=w304) -> (x/y=w305:cluster{"x":dbl, "y":dbl})
        n196 = case shown="1, Default" w315 {
          tunnel: [TRUE FALSE] -> w316
          frame 2 {
          }
          frame 1, Default {
          }
        }
        n197 = Divide(x=w305, y=w323) -> (x/y=w322:cluster{dbl, dbl})
        n198 = local write "image size [m]"(w305) -> ()
        n199 = local write "pixel size"(w322) -> ()
        n200 = local write "Bidirektional"(w316) -> ()
        n201 = Unbundle(w314) -> (w313:T25)  [unwired: 1 out]
        n202 = Index Array(array=w313, index=0 ("Index")) -> (element=w311:T26)
        n203 = Unbundle(w311) -> ("ROI Type"=w310:u32)  [unwired: 2 out]
        n204 = property on="Image" class="ImageControl"("ROI"=w314, "Current ROI Tool"=w310) -> ()  [unwired: 2 in, 2 out]
      }
      event "radius of view-x (6m)", "Galvo center [m] ii", "galvorotation (grad)": Value Change {
        w351 = TRUE  # flipy pixel is always 0 on top
        # "this has no objective magnification any more!"
        # "move this all to standard transform-parameters!"
        # "point (scansystem,m) for 00 (Pixel left top)"
        # "move image\nmove ROI"
        # "change image! (scale???)\nchange ROI! (scale have scan in shift register?)"
        n205 = event-data() -> ()  [unwired: 7 out]
        n206 = Negate(x="radius of view-x (6m)") -> (-x=w349:dbl)
        n207 = Select(t="radius of view-x (6m)", s=w351, f=w349) -> (s? t:f=w352:dbl)
        n208 = Unbundle(w346) -> ("Width"=w358:u32, "Height"=w361:u32)
        n209 = Divide(x=w361, y=w358) -> (x/y=w359:dbl)
        n210 = Multiply(x=w359, y=w352) -> (x*y=w360:dbl)
        n211 = Bundle(w349, w360) -> (w369:cluster{dbl, dbl})  [unwired: 1 out]
        n212 = Multiply(x="galvorotation (grad)", y=3.141592653589793) -> (x*y=w364:dbl)
        n213 = Divide(x=w364, y=180.0) -> (x/y=w353:dbl)
        n214 = Negate(x=w353) -> (-x=w355:dbl)
        n215 = call "VektorRotate.vi"("xyStart"=w369, "angel [rad]"=w355) -> ("rotated point"=w368:cluster{dbl, dbl})
        n216 = Add(x=w368, y="Galvo center [m] ii") -> (x+y=w348:cluster{dbl, dbl})
        n217 = Multiply(x=2.0, y="radius of view-x (6m)") -> (x*y=w347:dbl)
        n218 = local read "Transform"() -> (w366:T1)
        n219 = Divide(x=w358, y=w347) -> (x/y=w357:dbl)
        n220 = Bundle(cluster=w366, "00 Pixel [m]"=w348, "Rotate (rad)"=w353, "MirrorY"=w351, "pix/m"=w357) -> (w362:T1)
        n221 = local write "Transform"(w362) -> ()
      }
      event "Objektive": Value Change {
        # "modify field of view?\nWarning if scan too large?"
        n222 = event-data() -> ()  [unwired: 7 out]
        n223 = Number To Fractional String(use system decimal point (T)=FALSE, number="Objektive") -> (F-format string=w372:string)  [unwired: 2 out]
        n224 = Match Pattern(string=w372, regular expression="0*$") -> (before substring=w371:string)  [unwired: 4 out]
        n225 = call "Variables.vi"("value"=w371, "Tag in"="obj.mag", "Command"=T5."ChangeValue") -> ()  [unwired: 3 out]
      }
      event "Image": Mouse Up {
        # "pixel units.."
        n226 = event-data() -> ()  [unwired: 9 out]
        n227 = local read "Transform"() -> (w382:T1)
        n228 = local read "Objektive"() -> (w379:dbl)
        n229 = Unbundle By Name(w382) -> ("pix/m"=w381:dbl)
        n230 = local read "image size [m]"() -> (w384:cluster{"x":dbl, "y":dbl})
        n231 = Multiply(x=w381, y=w379) -> (x*y=w380:dbl)
        n232 = property on="Image" class="ImageControl"() -> ("ROI"=w389:T13)  [unwired: 2 in, 2 out]
        n233 = Multiply(x=w384, y=w380) -> (x*y=w383:cluster{"x":dbl, "y":dbl})
        n234 = call "ROItoFastSlow.vi"("ROI"=w389, "old fast slow (for y arb. scan only)"=w383) -> ("error out"=w386:errorcluster, "fast slow"=w387:cluster{"Vektorlänge":dbl, "Vektorlänge":dbl})
        n235 = case shown="No Error" w386 {
          tunnel: w387 -> [w392 _]
          tunnel: w385 -> [w391 _]
          tunnel: w380 -> [w390 _]
          frame No Error {
            n236 = flat-sequence {
              tunnel: w392 -> [w394]
              tunnel: w390 -> [w393]
              tunnel: w391 -> [w396]
              frame #0 {
                n237 = Divide(x=w394, y=w393) -> (x/y=w395:cluster{"Vektorlänge":dbl, "Vektorlänge":dbl})
                n238 = local write "image size [m]"(w395) -> ()
              }
              frame #1 {
                n239 = Generate User Event(user event=w396, event data cluster="update" ("event data")) -> ()  [unwired: 1 in, 2 out]
              }
            }
          }
          frame Error {
          }
        }
      }
      event "Image": Mouse Move {
        n240 = event-data() -> ()  [unwired: 6 out]
        n241 = local read "Transform"() -> (w401:T1)
        n242 = property on="Image" class="ImageControl"() -> ("Last Mouse Position"=w398:cluster{"X":i32, "Y":i32})  [unwired: 2 in, 2 out]
        n243 = call "xyCoordinateTransform.vi"("Point in"=w398, "Transform (Center first)"=w401, "Back"=TRUE) -> ("Point Out"=→"Galvo pos i.image [m]":cluster{dbl, dbl})  [unwired: 2 out]
      }
      event "image size [m]": Value Change {
        # "center"
        # "relative scaling"
        n244 = event-data() -> ("OldVal"=w433:cluster{"x":dbl, "y":dbl}, "NewVal"=w434:cluster{"x":dbl, "y":dbl})  [unwired: 5 out]
        n245 = Divide(x=w434, y=w433) -> (x/y=w408:cluster{"x":dbl, "y":dbl})
        n246 = property on="Image" class="ImageControl"() -> ("ROI"=w435:T13)  [unwired: 2 in, 2 out]
        n247 = Unbundle(w435) -> ("Global Rectangle"=w437:i32[], "Contours"=w425:T14)
        n248 = Generate User Event(user event=w403, event data cluster="update" ("event data")) -> ()  [unwired: 1 in, 2 out]
        n249 = Index Array(array=w425, index=0) -> (element=w406:T15)
        n250 = Array To Cluster(array=w437) -> (cluster=w436:T27)
        n251 = Unbundle(w406) -> ("ROI Type"=w424:u32, "Points"=w423:i32[])  [unwired: 1 out]
        n252 = Unbundle(w436) -> ("Global Rectangle[0]"=w431:i32, "Global Rectangle[1]"=w430:i32, "Global Rectangle[2]"=w429:i32, "Global Rectangle[3]"=w428:i32)
        n253 = Bundle("Global Rectangle[0]"=w431, "Global Rectangle[1]"=w430) -> (w412:T19)  [unwired: 1 out]
        n254 = Bundle("Global Rectangle[2]"=w429, "Global Rectangle[3]"=w428) -> (w411:T28)  [unwired: 1 out]
        n255 = Subtract(x=w411, y=w412) -> (x-y=w427:cluster{i32, i32})
        n256 = Divide(x=w427, y=2) -> (x/y=w420:cluster{dbl, dbl})
        n257 = Add(x=w412, y=w420) -> (x+y=w413:cluster{dbl, dbl})
        n258 = case shown="4" w424 {
          tunnel: w423 -> [w438 w439 w453 w483 w486]
          tunnel: [w438 w439 w440 w482 w490] -> w405
          tunnel: w413 -> [_ _ w448 w462 w492]
          tunnel: w408 -> [_ _ w449 w478 w493]
          frame 0, Default {
          }
          frame 1 {
            # "1 Point: 1.Array: x,y, 2.Array ignore"
          }
          frame 3, 12 {
            # "3,12 Type rect: \n2.array: xmin ymin xmax ymax rotation(grad*1000)"
            n259 = Array To Cluster(array=w453) -> (cluster=w458:T29)
            n260 = Unbundle(w458) -> ("Points[0]"=w457:i32, "Points[1]"=w456:i32, "Points[2]"=w455:i32, "Points[3]"=w454:i32, "Points[4]"=w445:i32)
            n261 = Bundle("Points[0]"=w457, "Points[1]"=w456) -> (w451:cluster{"Points[0]":i32, "Points[1]":i32})  [unwired: 1 out]
            n262 = Bundle("Points[2]"=w455, "Points[3]"=w454) -> (w450:cluster{"Points[2]":i32, "Points[3]":i32})  [unwired: 1 out]
            n263 = call "ScalePoint.vi"("Scaling"=w449, "Center"=w448, "Point"=w451) -> ("new Point"=w447:cluster{dbl, dbl})
            n264 = call "ScalePoint.vi"("Scaling"=w449, "Center"=w448, "Point"=w450) -> ("new Point"=w446:cluster{dbl, dbl})
            n265 = Unbundle(w447) -> (w444:dbl, w443:dbl)
            n266 = Unbundle(w446) -> (w442:dbl, w441:dbl)
            n267 = Build Array(w444, w443, w442, w441, w445) -> (w452:dbl[])
            n268 = To Long Integer(number=w452) -> (32bit integer=w440:i32[])
          }
          frame 4 {
            # "length"
            # "find changed"
            # "oval should be circle"
            n269 = Unbundle(w478) -> ("x"=w480:dbl, "y"=w479:dbl)
            n270 = Array To Cluster(array=w483) -> (cluster=w485:T30)
            n271 = Unbundle(w485) -> ("Points[0]"=w474:i32, "Points[1]"=w475:i32, "Points[2]"=w476:i32, "Points[3]"=w477:i32)
            n272 = call "equal_real.vi"("b"=1.0, "a"=w479) -> ("Equal"=w471:bool)  [unwired: 1 in]
            n273 = Subtract(x=w476, y=w474) -> (x-y=w473:i32)
            n274 = Subtract(x=w477, y=w475) -> (x-y=w472:i32)
            n275 = Select(t=w480, s=w471, f=w479) -> (s? t:f=w467:dbl)
            n276 = Select(t=w473, s=w471, f=w472) -> (s? t:f=w470:i32)
            n277 = Divide(x=w470, y=2) -> (x/y=w468:dbl)
            n278 = Multiply(x=w468, y=w467) -> (x*y=w463:dbl)
            n279 = Subtract(x=w462, y=w463) -> (x-y=w466:cluster{dbl, dbl})
            n280 = Add(x=w462, y=w463) -> (x+y=w461:cluster{dbl, dbl})
            n281 = Unbundle(w461) -> (w460:dbl, w459:dbl)
            n282 = Unbundle(w466) -> (w465:dbl, w464:dbl)
            n283 = Build Array(w465, w464, w460, w459) -> (w484:dbl[])
            n284 = To Long Integer(number=w484) -> (32bit integer=w482:i32[])
          }
          frame 10 {
            # "only use x"
            # "10 Line,polyline: 2.array: yx,yx,yx,yx...,xy-increment"
            n285 = Unbundle(w493) -> ("x"=w487:dbl)  [unwired: 1 out]
            n286 = Type Cast(type=cluster{i32, i32}[] [], x=w486) -> (*(type *) &x=w494:cluster{i32, i32}[])
            n287 = Bundle("x"=w487, "x"=w487) -> (w488:cluster{"x":dbl, "x":dbl})  [unwired: 1 out]
            n288 = for {
              tunnel: w494 -> [w499] mode=indexing
              tunnel: w488 -> [w498]
              tunnel: w492 -> [w497]
              tunnel: [w496] -> w491 mode=indexing
              n289 = call "ScalePoint.vi"("Scaling"=w498, "Center"=w497, "Point"=w499) -> ("new Point"=w496:cluster{dbl, dbl})
            }
            n290 = To Long Integer(number=w491) -> (32bit integer=w489:cluster{i32, i32}[])
            n291 = Type Cast(type=w486, x=w489) -> (*(type *) &x=w490:i32[])
          }
        }
        n292 = call "ScalePoint.vi"("Scaling"=w408, "Center"=w413, "Point"=w411) -> ("new Point"=w409:cluster{dbl, dbl})
        n293 = call "ScalePoint.vi"("Scaling"=w408, "Center"=w413, "Point"=w412) -> ("new Point"=w410:cluster{dbl, dbl})
        n294 = Unbundle(w410) -> (w419:dbl, w418:dbl)
        n295 = Unbundle(w409) -> (w417:dbl, w416:dbl)
        n296 = Build Array(w419, w418, w417, w416) -> (w415:dbl[])
        n297 = To Long Integer(number=w415) -> (32bit integer=w414:i32[])
        n298 = Bundle(cluster=w406, "Points"=w405) -> (w407:T15)  [unwired: 2 out]
        n299 = Build Array(w407) -> (w422:T14)
        n300 = Bundle(w414, w422) -> (w421:T31)  [unwired: 1 out]
        n301 = property on="Image" class="ImageControl"("ROI"=w421) -> ()  [unwired: 2 in, 2 out]
      }
      event "pixel size": Value Change {
        # "change pixels"
        n302 = event-data() -> ("NewVal"=w502:cluster{dbl, dbl})  [unwired: 6 out]
        n303 = flat-sequence {
          tunnel: w502 -> [w512]
          tunnel: w501 -> [w519]
          frame #0 {
            w509 = cluster{i32, i32} {1, 2}
            # "if 0/0 reuse old"
            n304 = local read "image size [m]"() -> (w513:cluster{"x":dbl, "y":dbl})
            n305 = Divide(x=w513, y=w512) -> (x/y=w504:cluster{dbl, dbl})
            n306 = Unbundle(w504) -> (w505:dbl)  [unwired: 1 out]
            n307 = Equal?(x=w505, y=inf) -> (x = y?=w507:bool)
            n308 = case shown="False" w507 {
              tunnel: w504 -> [w514 w518]
              tunnel: [w514 w517] -> w503
              frame False {
              }
              frame True {
                n309 = local read "pixels"() -> (w515:cluster{"x-Pixel":i32, "y-Pixel":u16})
                n310 = Unbundle(w515) -> ("y-Pixel"=w516:u16)  [unwired: 1 out]
                n311 = Bundle(cluster=w518, w516) -> (w517:cluster{dbl, dbl})  [unwired: 1 out]
              }
            }
            n312 = Divide(x=w503, y=w509) -> (x/y=w511:cluster{dbl, dbl})
            n313 = To Long Integer(number=w511) -> (32bit integer=w510:cluster{i32, i32})
            n314 = Multiply(x=w510, y=w509) -> (x*y=w508:cluster{i32, i32})
            n315 = local write "pixels"(w508) -> ()
          }
          frame #1 {
            n316 = Generate User Event(user event=w519, event data cluster="update" ("event data")) -> ()  [unwired: 1 in, 2 out]
          }
        }
      }
      event "pixels": Value Change {
        n317 = event-data() -> ("NewVal"=w525:cluster{"x-Pixel":i32, "y-Pixel":u16})  [unwired: 6 out]
        n318 = Generate User Event(user event=w521, event data cluster="update" ("event data")) -> ()  [unwired: 1 in, 2 out]
        n319 = local read "image size [m]"() -> (w526:cluster{"x":dbl, "y":dbl})
        n320 = Divide(x=w526, y=w525) -> (x/y=w524:cluster{dbl, dbl})
        n321 = local write "pixel size"(w524) -> ()
      }
      event "experiment": Value Change {
        n322 = event-data() -> ()  [unwired: 7 out]
        n323 = call "Variables.vi"("value"="experiment", "Tag in"="experiment", "Command"=T5."ChangeValue") -> ()  [unwired: 3 out]
      }
      event "Exit": Value Change {
        n324 = event-data() -> ()  [unwired: 7 out]
        n325 = case shown="False" "do not close at end" {
          frame False {
            n326 = invoke class="VI" method="FP.Close"() -> ()  [unwired: 3 in, 3 out]
          }
          frame True {
          }
        }
      }
      event "time [s]/point": Value Change; User Event {
        n327 = event-data() -> ()  [unwired: 4 out]
        n328 = local read "image size [m]"() -> (w533:cluster{"x":dbl, "y":dbl})
        n329 = local read "keep const."() -> (w534:u16)
        n330 = case shown="0, Default" w534 {
          tunnel: w533 -> [w550 w558]
          tunnel: [w545 w556] -> w532
          frame 0, Default {
            w546 = cluster{i32, i32} {1, 2}
            # "if 0/0 reuse old"
            # "x: multiple of 1\ny: multiple of 2"
            # "pix size"
            n331 = local read "pixel size"() -> (w549:cluster{dbl, dbl})
            n332 = Divide(x=w550, y=w549) -> (x/y=w543:cluster{dbl, dbl})
            n333 = Unbundle(w543) -> (w542:dbl)  [unwired: 1 out]
            n334 = Equal?(x=w542, y=inf) -> (x = y?=w540:bool)
            n335 = case shown="True" w540 {
              tunnel: w543 -> [w551 w555]
              tunnel: [w551 w554] -> w544
              frame False {
              }
              frame True {
                n336 = local read "pixels"() -> (w553:cluster{"x-Pixel":i32, "y-Pixel":u16})
                n337 = Unbundle(w553) -> ("y-Pixel"=w552:u16)  [unwired: 1 out]
                n338 = Bundle(cluster=w555, w552) -> (w554:cluster{dbl, dbl})  [unwired: 1 out]
              }
            }
            n339 = Divide(x=w544, y=w546) -> (x/y=w548:cluster{dbl, dbl})
            n340 = To Long Integer(number=w548) -> (32bit integer=w547:cluster{i32, i32})
            n341 = Multiply(x=w547, y=w546) -> (x*y=w545:cluster{i32, i32})
            n342 = local write "pixels"(w545) -> ()
          }
          frame 1 {
            # "Pixels"
            n343 = local read "pixels"() -> (w556:cluster{"x-Pixel":i32, "y-Pixel":u16})
            n344 = Divide(x=w558, y=w556) -> (x/y=w557:cluster{dbl, dbl})
            n345 = local write "pixel size"(w557) -> ()
          }
        }
        n346 = Unbundle(w532) -> ("x-Pixel"=w536:i32, "y-Pixel"=w535:i32)
        n347 = Compound Arithmetic op=MULTIPLY("time [s]/point", w536, w535) -> (→"total time [s]":dbl)
      }
    }
  }
  n348 = Unregister For Events(event registration refnum=w37) -> ()  [unwired: 1 in, 1 out]
